vi "TDMS In Memory Read from Network.vi"() -> ()   [LabVIEW 2023]
doc: "This example demonstrates how to read data from a network .tdms file using the TDMS In Memory functions."
panel:
  out "File Size (byte)":i64
  out "Waveform Graph":waveform(dbl)(graph)
  # "Overview: Demonstrates the use of the TDMS In Memory functions to read a .tdms file from network.\nInstructions:\n1. Run the TDMS In Memory Write to Network.vi before running this VI.\n2. Run this VI. Waveform Graph displays the data of the .tdms file in memory read from the network. File Size (byte) returns the size of the .tdms file in memory.\n3. Delete the TDMS file (located at  [LabVIEW Data]\\Example TDMS In Memory From Network.tdms) when you are done."
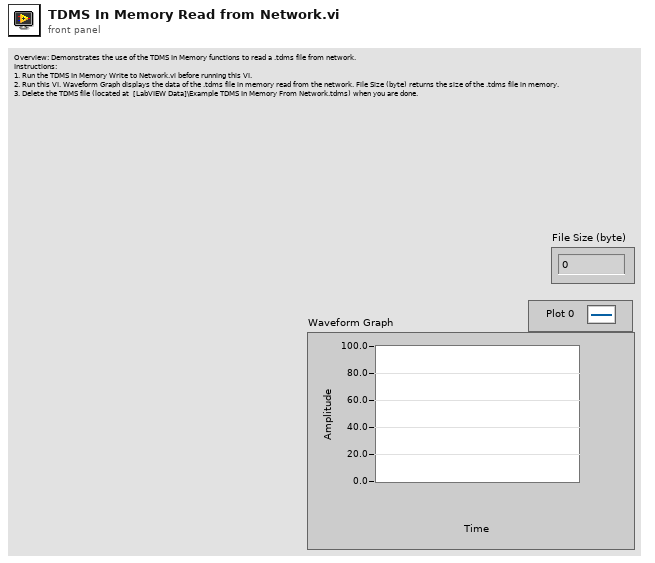
[diagram p1: front panel]
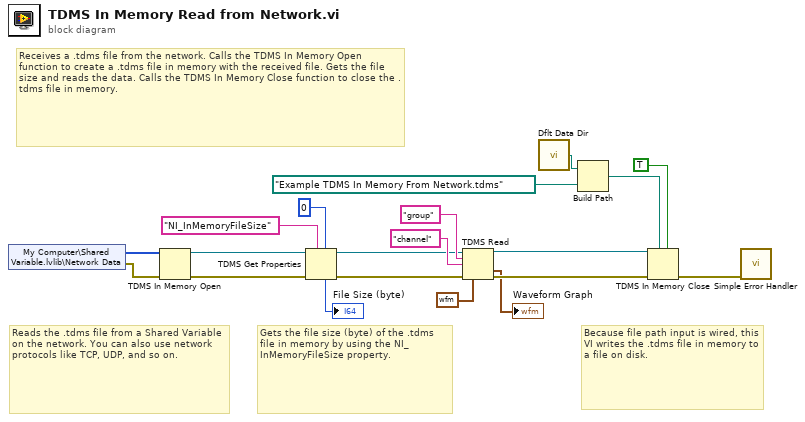
[diagram p0: block diagram]
diagram:
  # "Gets the file size (byte) of the .tdms file in memory by using the NI_InMemoryFileSize property."
  # "Reads the .tdms file from a Shared Variable on the network. You can also use network protocols like TCP, UDP, and so on."
  # "Because file path input is wired, this VI writes the .tdms file in memory to a file on disk."
  # "Receives a .tdms file from the network. Calls the TDMS In Memory Open function to create a .tdms file in memory with the received file. Gets the file size and reads the data. Calls the TDMS In Memory Close function to close the .tdms file in memory."
  n1 = shared-variable "My Computer\\Shared Variable.lvlib\\Network Data"() -> (w9:u8[], error out=w1:errorcluster)  [unwired: 1 in]
  n2 = TDMS In Memory Open(8:w1, 11:w9) -> (0:w12:errorcluster, 3:w13:refnum<k34>)
  n3 = TDMS Get Properties(5:i64 0, 7:"NI_InMemoryFileSize" ("property name"), 8:w12, 11:w13) -> (0:w10:errorcluster, 3:w11:refnum<k34>, 4:→"File Size (byte)":i64)  [unwired: 2 in, 3 out]
  n4 = TDMS Read(0:w11, 5:"group" ("group name in"), 7:"channel", 11:w10, 12:waveform(dbl) {"t0"=timestamp(0 s since 1904-01-01), "dt"=1.0, "Y"=[]} ("output waveform")) -> (4:w19:refnum<k34>, 10:→"Waveform Graph":waveform(dbl), 15:w18:errorcluster)  [unwired: 3 in, 3 out]
  n5 = call <vilib>:"Dflt Data Dir.vi"() -> ("App:Default Data Directory"=w5:path)
  n6 = Build Path(base path=w5, name or relative path=path "Example TDMS In Memory From Network.tdms") -> (appended path=w3:path)
  n7 = TDMS In Memory Close(5:TRUE ("overwrite (F)"), 7:w3, 8:w18, 11:w19) -> (0:w20:errorcluster)
  n8 = call <vilib>:"Simple Error Handler.vi"("error in (no error)"=w20) -> ()  [unwired: 4 in, 5 out]
